vi "Actor Core.vi"(8 "error in":errorcluster, 11 "Report Viewer in":refnum<class "Report Viewer.lvclass">) -> (0 "error out":errorcluster, 3 "Actor out":refnum<class "Actor.lvclass">)   [LabVIEW 2019, in "Report Viewer.lvlib" / "Report Viewer.lvclass"]
doc: "The user interface for this panel.\n\n----\nPlease see the following web address for additional documentation and tutorial information:\nhttp://www.mooregoodideas.com/mgi-panel-manager/\n\nAuthor: Derek Trepanier\n\nCopyright (c) 2018, Moore Good Ideas, Inc.\n\nAll rights reserved.\n\nRedistribution and use in source and binary forms, with or without modification, are permitted provided that the following conditions are met:\n\n * Redistributions of source code must retain the above copyright notice, this list of conditions and the following disclaimer.\n * Redistributions in binary form must reproduce the above copyright notice, this list of conditions and the following disclaimer in the documentation and/or other materials provided with the distribution.\n * Neither the name of Moore Good Ideas, Inc. nor the names of its contributors may be used to endorse or promote products derived from this software without specific prior written permission.\n\nTHIS SOFTWARE IS PROVIDED BY THE COPYRIGHT HOLDERS AND CONTRIBUTORS \"AS IS\" AND ANY EXPRESS OR IMPLIED WARRANTIES, INCLUDING, BUT NOT LIMITED TO, THE IMPLIED WARRANTIES OF MERCHANTABILITY AND FITNESS FOR A PARTICULAR PURPOSE ARE DISCLAIMED. IN NO EVENT SHALL THE COPYRIGHT OWNER OR CONTRIBUTORS BE LIABLE FOR ANY DIRECT, INDIRECT, INCIDENTAL, SPECIAL, EXEMPLARY, OR CONSEQUENTIAL DAMAGES (INCLUDING, BUT NOT LIMITED TO, PROCUREMENT OF SUBSTITUTE GOODS OR SERVICES; LOSS OF USE, DATA, OR PROFITS; OR BUSINESS INTERRUPTION) HOWEVER CAUSED AND ON ANY THEORY OF LIABILITY, WHETHER IN CONTRACT, STRICT LIABILITY, OR TORT (INCLUDING NEGLIGENCE OR OTHERWISE) ARISING IN ANY WAY OUT OF THE USE OF THIS SOFTWARE, EVEN IF ADVISED OF THE POSSIBILITY OF SUCH DAMAGE."
uses:
  Library/Report Viewer.lvclass
  builds/Engine/Actor Framework.lvlibp/1abvi3w/vi.lib/ActorFramework/Actor/Actor.lvclass
  Library/Report Viewer.lvclass/Report Viewer.ctl
  Report Viewer Messages/Update From Selection Msg/Update From Selection Msg.lvclass/Update From Selection Msg.ctl
  Report Viewer Messages/Write Data Start Time Msg/Write Data Start Time Msg.lvclass/Write Data Start Time Msg.ctl
  Accessors/Write Filename_ref.vi
  Accessors/GUI/Write Tree Refnum.vi
  Accessors/GUI/Write Graph_Ref.vi
  Accessors/GUI/Write Properties_Ref.vi
  Accessors/GUI/Write Values_Ref.vi
  Private/Tree/Clear Tree.vi
  builds/Engine/Actor Framework.lvlibp/1abvi3w/vi.lib/ActorFramework/Message Enqueuer/Enqueue.vi
  Report Viewer Messages/Open Report Msg/Open Report Msg.lvclass
  Report Viewer Messages/Update From Selection Msg/Update From Selection Msg.lvclass
  Report Viewer Messages/File Settings Dialog Msg/File Settings Dialog Msg.lvclass
  Report Viewer Messages/Write Data Start Time Msg/Write Data Start Time Msg.lvclass
  builds/Base Software/Panels/Prime Panel.lvlibp/Project/Prime Panel.lvclass
panel:
  in  "File contents":string[](tree)
  out "File Name":string
  in  "Settings":bool
  in  "Open TDMS":bool
  in  "Tab Control":T1(tab)
  in  "Properties Table":i32(listbox)
  in  "Values Table":i32(listbox)
  out "Waveform Graph":waveform(dbl)[](graph)
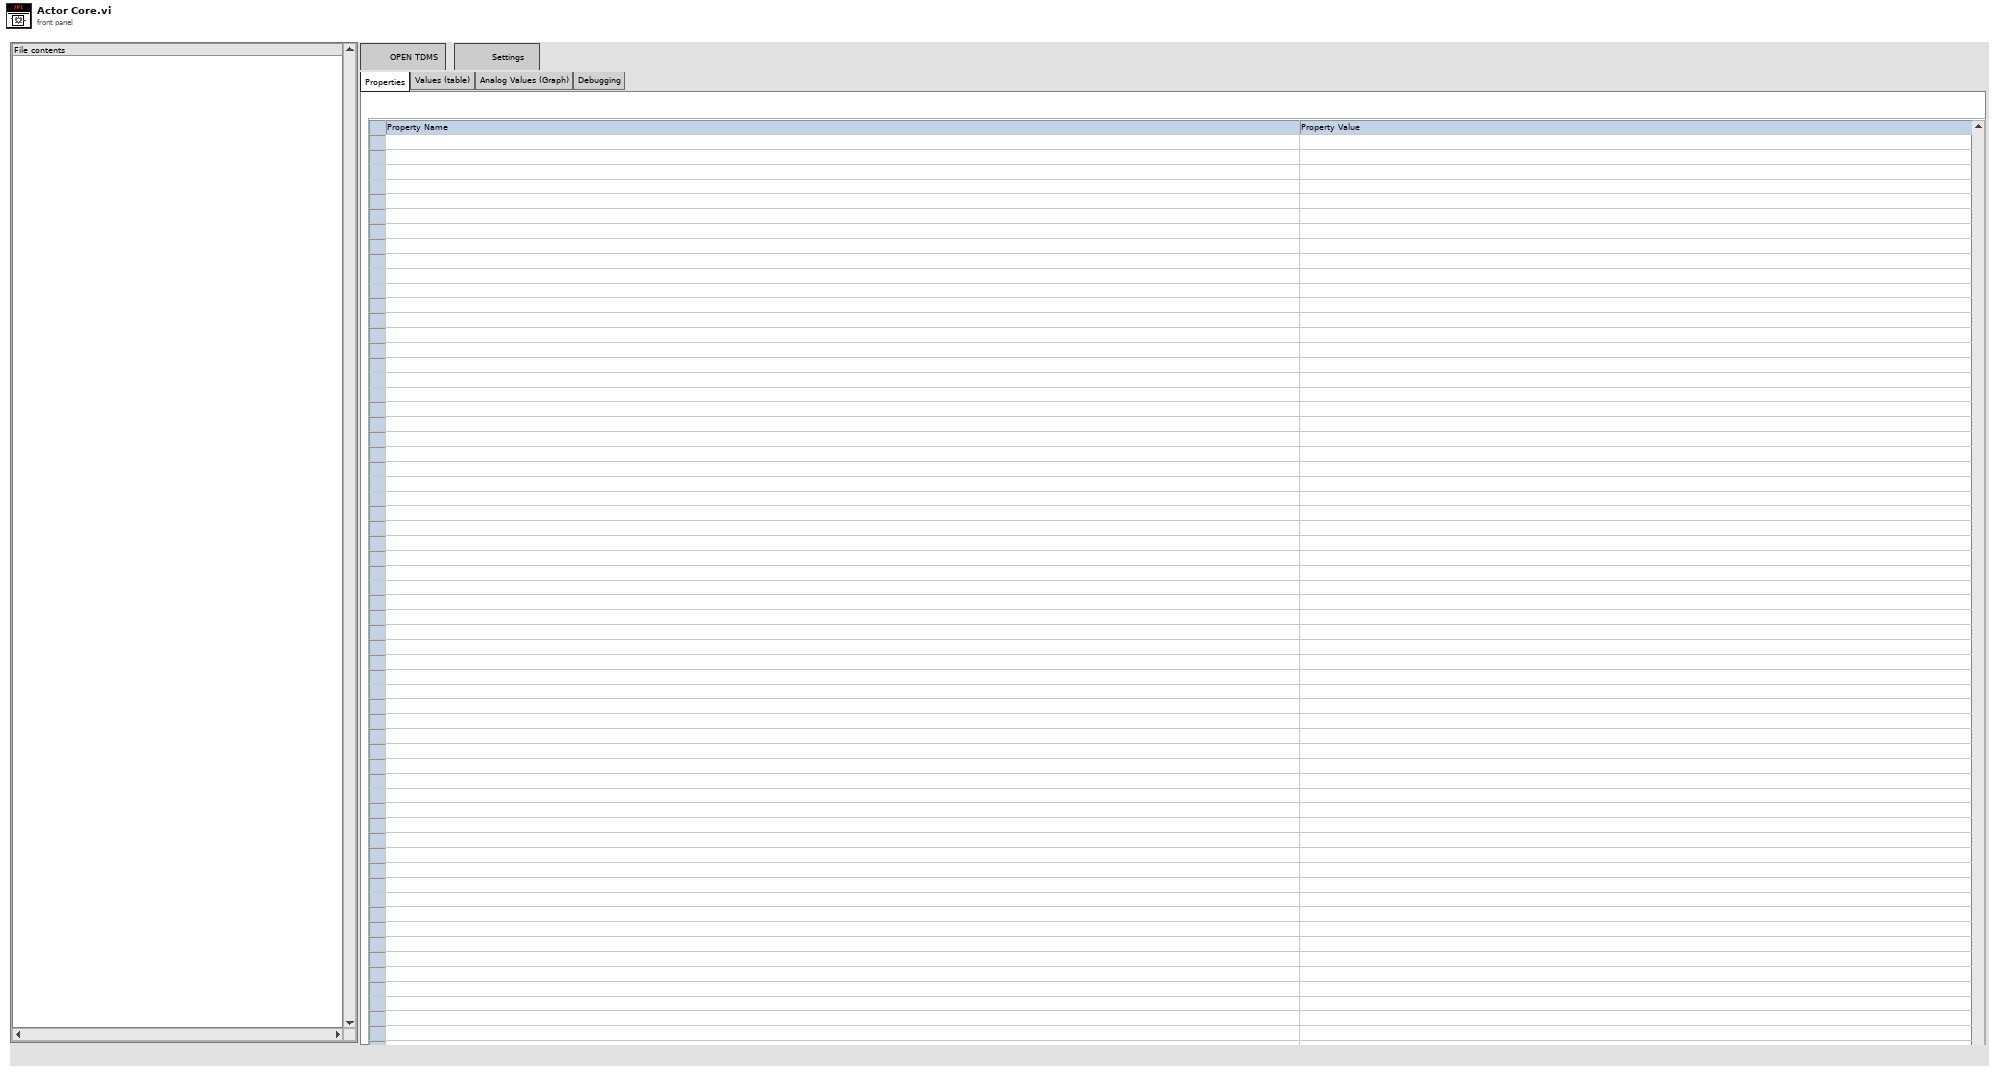
[diagram p1: front panel]
types:
  T1 = enum32{"Properties", "Values (table)", "Analog Values (Graph)", "Debugging"}
  T2 = cluster{"Pnl Actor":refnum<event-registration>, "Event Registration Refnum":refnum<event-registration>}
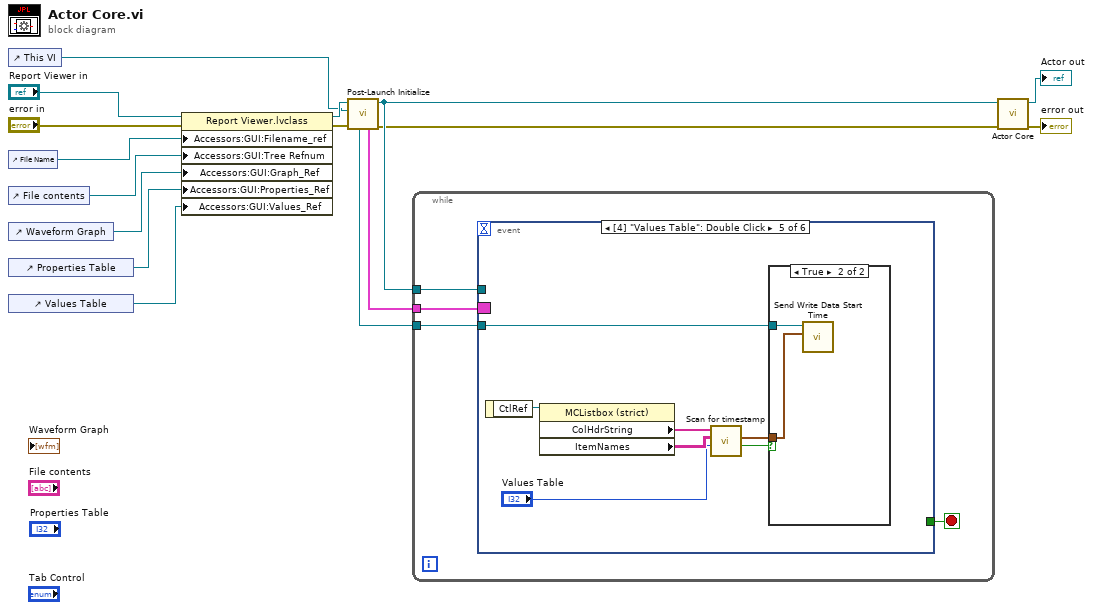
[diagram p0: block diagram]
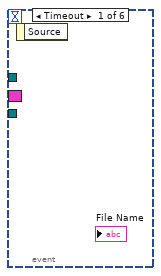
[diagram p2: hidden frame]
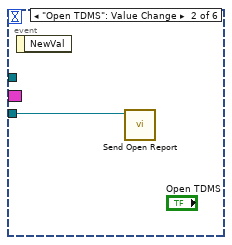
[diagram p3: hidden frame]
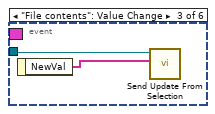
[diagram p4: hidden frame]
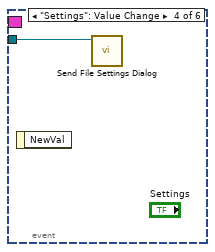
[diagram p5: hidden frame]
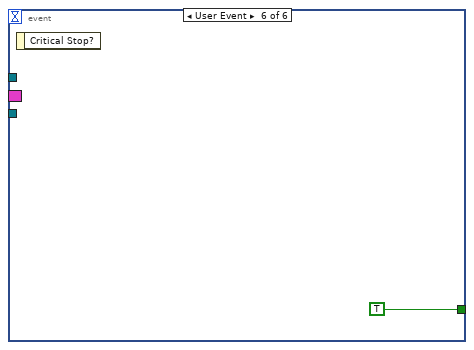
[diagram p7: hidden frame]
diagram:
  n1 = control-ref of="This VI"() -> (w6:refnum<vi>)
  n2 = control-ref of="File Name"() -> (w5:refnum<vi>)
  n3 = control-ref of="File contents"() -> (w4:refnum<vi>)
  n4 = control-ref of="Waveform Graph"() -> (w3:refnum<vi>)
  n5 = control-ref of="Properties Table"() -> (w2:refnum<vi>)
  n6 = control-ref of="Values Table"() -> (w1:refnum<vi>)
  n7 = property class="Report Viewer.lvclass"(reference="Report Viewer in", error in="error in", "Accessors:GUI:Filename_ref"=w5, "Accessors:GUI:Tree Refnum"=w4, "Accessors:GUI:Graph_Ref"=w3, "Accessors:GUI:Properties_Ref"=w2, "Accessors:GUI:Values_Ref"=w1) -> (reference out=w7:refnum<class "Report Viewer.lvclass">, error out=w8:errorcluster)
  n8 = call "Post-Launch Initialize.vi"("error in"=w8, "GUI_Ref"=w6, "Report Viewer in"=w7) -> ("error out"=w13:errorcluster, "Report Viewer out"=w14:refnum<class "Report Viewer.lvclass">, "Registered Events"=w12:T2, "Self Enqueuer"=w11:refnum<class "Message Enqueuer.lvclass">)  [unwired: 5 in]
  n9 = while {
    tunnel: w12 -> [w20]
    tunnel: w11 -> [w19]
    tunnel: w14 -> [w18]
    stop <- w17 stop-if-true
    n10 = event shown="[4] \"Values Table\": Double Click" {
      selector: w20 -> [_ _ _ _ _ _]
      dyn-events: _ -> [_ _ _ _ _ _]
      timeout: _ -> [_ _ _ _ _ _]
      tunnel: w19 -> [_ w21 w23 w24 w26 _]
      tunnel: w18 -> [_ _ _ _ _ _]
      tunnel: [_ _ _ _ _ TRUE] -> w17
      event Timeout {
        n11 = event-data() -> ()  [unwired: 1 in, 1 out]
      }
      event "Open TDMS": Value Change {
        n12 = event-data() -> ()  [unwired: 1 in, 1 out]
        n13 = call "Send Open Report.vi"("Message Enqueuer"=w21) -> ()  [unwired: 9 in, 2 out]
      }
      event "File contents": Value Change {
        n14 = event-data() -> ("NewVal"=w22:string[])  [unwired: 1 in]
        n15 = call "Send Update From Selection.vi"("File Contents"=w22, "Message Enqueuer"=w23) -> ()  [unwired: 8 in, 2 out]
      }
      event "Settings": Value Change {
        n16 = event-data() -> ()  [unwired: 1 in, 1 out]
        n17 = call "Send File Settings Dialog.vi"("Message Enqueuer"=w24) -> ()  [unwired: 9 in, 2 out]
      }
      event "Values Table": Double Click {
        n18 = event-data() -> ("CtlRef"=w31:refnum<vi>)  [unwired: 1 in]
        n19 = property class="MCListbox (strict)"(reference=w31) -> ("ColHdrString"=w30:string[], "ItemNames"=w29:string[][])  [unwired: 1 in, 2 out]
        n20 = call "Scan for timestamp.vi"("Row Index"="Values Table", "Item Names"=w29, "Column Headers"=w30) -> ("found"=w27:bool, "Time Stamp"=w25:timestamp)  [unwired: 7 in]
        n21 = case shown="True" w27 {
          tunnel: w26 -> [_ w33]
          tunnel: w25 -> [_ w32]
          frame False {
          }
          frame True {
            n22 = call "Send Write Data Start Time.vi"("Data Start Time"=w32, "Message Enqueuer"=w33) -> ()  [unwired: 8 in, 2 out]
          }
        }
      }
      event User Event {
        n23 = event-data() -> ()  [unwired: 1 in, 1 out]
      }
    }
  }
  n24 = call-parent "Actor Core.vi"("error in"=w13, "Prime Panel in"=w14) -> ("error out"=→"error out":errorcluster, "Actor out"=→"Actor out":refnum<class "Actor.lvclass">)  [unwired: 8 in]
